vi "rqcAlice ServiceNET Read Command.vi"(8 "error in":errorcluster, 11 "rqcAlice ServiceNET in":T2) -> (0 "error out":errorcluster, 1 "cmd valid":bool, 2 "command":T1, 3 "rqcAlice ServiceNET out":T2)   [LabVIEW 2018]
uses:
  Custom Controls/rqcAlice ServiceNET control.ctl
  Custom Controls/rqc ServiceNET command.ctl
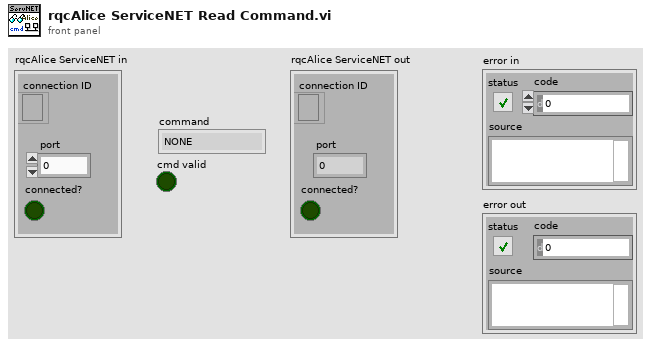
[diagram p1: front panel]
types:
  T1 = typedef "rqc ServiceNET command.ctl" = enum8{"NONE", "READY", "START", "PING", "SEND KEY", "WRITE KEY", "WRITE AND SAVE KEY"}
  T2 = typedef "rqcAlice ServiceNET control.ctl" = cluster{"connection ID":refnum<k5>, "port":u16, "connected?":bool}
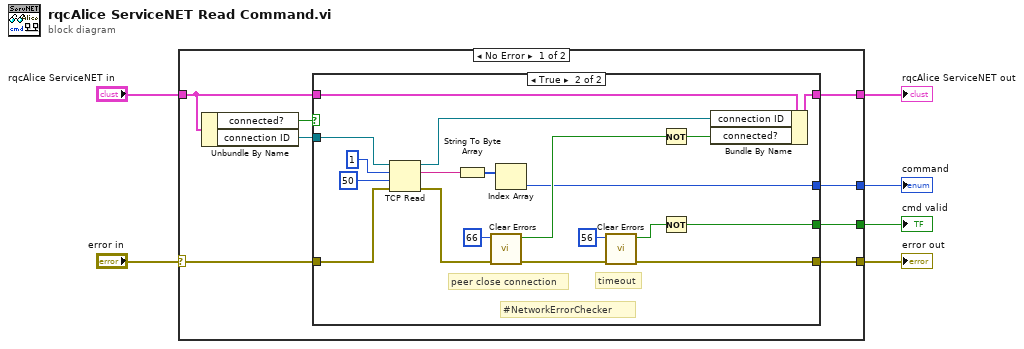
[diagram p0: block diagram]
diagram:
  n1 = case shown="No Error" "error in" {
    selector: "error in" -> [w10 w37]
    tunnel: [w9 w37] -> w5
    tunnel: "rqcAlice ServiceNET in" -> [w13 w36]
    tunnel: [w12 w36] -> w3
    tunnel: [w8 _] -> w2
    tunnel: [w7 _] -> w1
    frame No Error {
      n2 = Unbundle By Name(w13) -> ("connected?"=w14:bool, "connection ID"=w11:refnum<k5>)
      n3 = case shown="True" w14 {
        tunnel: [w16 w34] -> w12
        tunnel: w13 -> [w16 w35]
        tunnel: w11 -> [_ w31]
        tunnel: w10 -> [w15 w29]
        tunnel: [w15 w19] -> w9
        tunnel: [_ w24] -> w8
        tunnel: [_ w17] -> w7
        frame False {
        }
        frame True {
          # "peer close connection"
          # "timeout"
          # "#NetworkErrorChecker"
          n4 = TCP Read(connection ID=w31, bytes to read=1, error in (no error)=w29, 9:50 ("timeout ms (25000)")) -> (connection ID out=w30:refnum<k5>, data out=w25:string, error out=w21:errorcluster)  [unwired: 1 in]
          n5 = String To Byte Array(string=w25) -> (unsigned byte array=w26:u8[])
          n6 = call <vilib>:"Clear Errors.vi"("error in (no error)"=w21, "specific error code to clear (0: all)"=66) -> ("error out"=w20:errorcluster, "specific error cleared?"=w32:bool)  [unwired: 4 in]
          n7 = Index Array(array=w26) -> (element=w24:u8)  [unwired: 1 in]
          n8 = call <vilib>:"Clear Errors.vi"("error in (no error)"=w20, "specific error code to clear (0: all)"=56) -> ("error out"=w19:errorcluster, "specific error cleared?"=w18:bool)  [unwired: 4 in]
          n9 = Not(x=w32) -> (.not. x?=w33:bool)
          n10 = Not(x=w18) -> (.not. x?=w17:bool)
          n11 = Bundle By Name(cluster=w35, "connection ID"=w30, "connected?"=w33) -> (w34:T2)
        }
      }
    }
    frame Error {
    }
  }
  "rqcAlice ServiceNET out" <- w3
  "error out" <- w5
  "command" <- w2
  "cmd valid" <- w1
